vi "Force Array To Size.vi"(5 "Default Value":dbl format="%.2f", 6 "Boolean Array In":bool[](array[boolean]), 7 "# Elements":i32, 9 "2D U8 Array In":u8[][](array[numeric]), 10 "DBL Array In":dbl[](array[numeric]) format="%.2f", 11 "I32 Array In":i32[](array[numeric])) -> (1 "2D U8 Array Out":u8[][](array[numeric]), 2 "DBL Array Out":dbl[](array[numeric]) format="%.2f", 3 "I32 Array Out":i32[](array[numeric]), 4 "Boolean Array Out":bool[](array[boolean]))   [LabVIEW 2014]
panel:
  # "If input array has the specified number of elements, it is not changed.\nIf input array has more than the specified number of elements, the extra elements are removed from the end.\nIf input array has less than specified number of elements, it is padded using the default value."
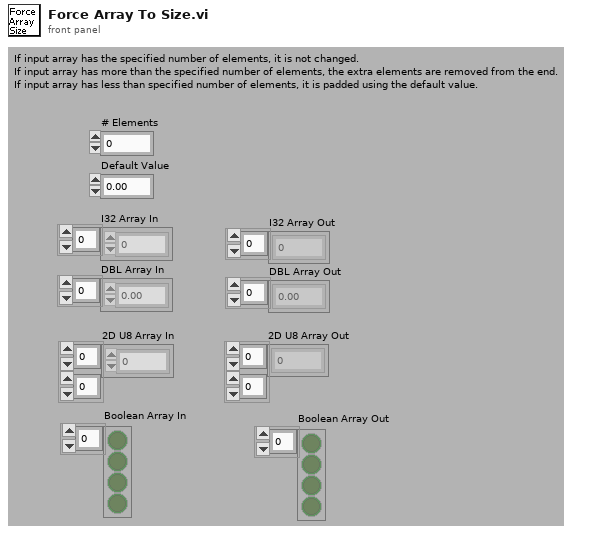
[diagram p1: front panel]
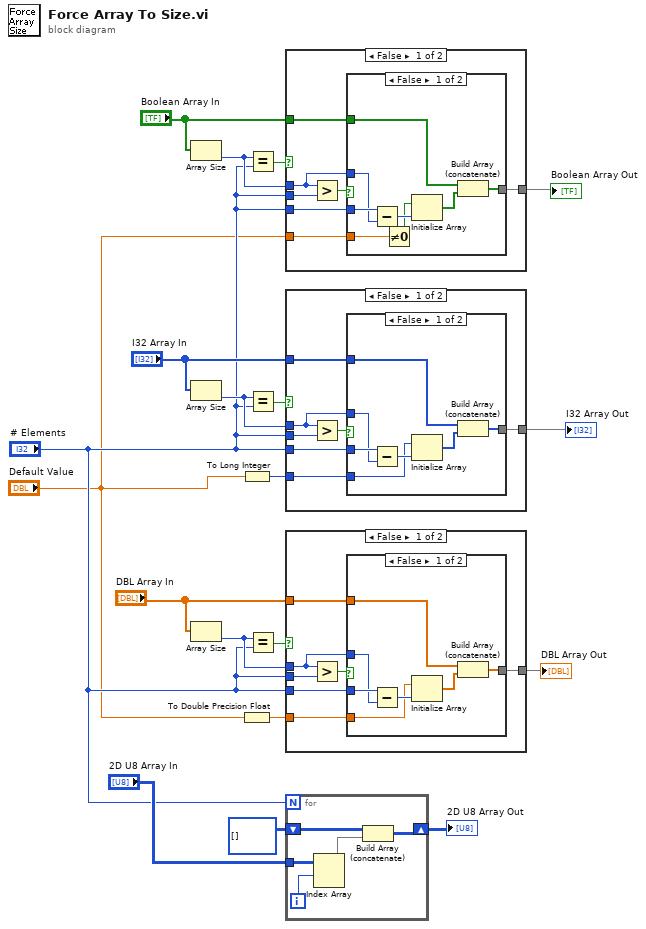
[diagram p0: block diagram]
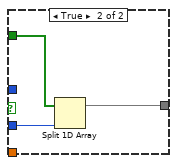
[diagram p2: hidden frame]
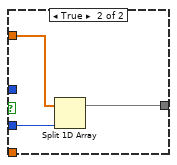
[diagram p4: hidden frame]
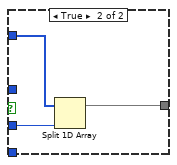
[diagram p6: hidden frame]
diagram:
  n1 = Array Size(array="Boolean Array In") -> (size(s)=w5:i32)
  n2 = Array Size(array="I32 Array In") -> (size(s)=w19:i32)
  n3 = Array Size(array="DBL Array In") -> (size(s)=w12:i32)
  n4 = To Long Integer(number="Default Value") -> (32bit integer=w16:i32)
  n5 = To Double Precision Float(number="Default Value") -> (double precision float=w14:dbl)
  n6 = Equal?(x=w5, y="# Elements") -> (x = y?=w6:bool)
  n7 = Equal?(x=w19, y="# Elements") -> (x = y?=w18:bool)
  n8 = Equal?(x=w12, y="# Elements") -> (x = y?=w13:bool)
  n9 = case shown="False" w6 {
    tunnel: w5 -> [w21 _]
    tunnel: "# Elements" -> [w26 _]
    tunnel: "# Elements" -> [w24 _]
    tunnel: "Boolean Array In" -> [w23 w38]
    tunnel: [w22 w38] -> w1
    tunnel: "Default Value" -> [w20 _]
    frame False {
      n10 = Greater?(x=w21, y=w26) -> (0:w25:bool)
      n11 = case shown="False" w25 {
        tunnel: w24 -> [w34 w37]
        tunnel: w23 -> [w30 w36]
        tunnel: [w29 w35] -> w22
        tunnel: w21 -> [w33 _]
        tunnel: w20 -> [w28 _]
        frame False {
          n12 = Subtract(x=w34, y=w33) -> (x-y=w32:i32)
          n13 = Not Equal To 0?(x=w28) -> (x != 0?=w27:bool)
          n14 = Initialize Array(w27, w32) -> (w31:bool[])
          n15 = Build Array (concatenate)(w30, w31) -> (w29:bool[])
        }
        frame True {
          n16 = Split 1D Array(array=w36, index=w37) -> (first subarray=w35:bool[])  [unwired: 1 out]
        }
      }
    }
    frame True {
    }
  }
  "Boolean Array Out" <- w1
  n17 = case shown="False" w18 {
    tunnel: w19 -> [w40 _]
    tunnel: "# Elements" -> [w45 _]
    tunnel: "# Elements" -> [w43 _]
    tunnel: "I32 Array In" -> [w42 w56]
    tunnel: [w41 w56] -> w15
    tunnel: w16 -> [w39 _]
    frame False {
      n18 = Greater?(x=w40, y=w45) -> (0:w44:bool)
      n19 = case shown="False" w44 {
        tunnel: w43 -> [w52 w55]
        tunnel: w42 -> [w47 w54]
        tunnel: [w46 w53] -> w41
        tunnel: w40 -> [w51 _]
        tunnel: w39 -> [w49 _]
        frame False {
          n20 = Subtract(x=w52, y=w51) -> (x-y=w50:i32)
          n21 = Initialize Array(w49, w50) -> (w48:i32[])
          n22 = Build Array (concatenate)(w47, w48) -> (w46:i32[])
        }
        frame True {
          n23 = Split 1D Array(array=w54, index=w55) -> (first subarray=w53:i32[])  [unwired: 1 out]
        }
      }
    }
    frame True {
    }
  }
  "I32 Array Out" <- w15
  n24 = case shown="False" w13 {
    tunnel: w12 -> [w58 _]
    tunnel: "# Elements" -> [w63 _]
    tunnel: "# Elements" -> [w61 _]
    tunnel: "DBL Array In" -> [w60 w74]
    tunnel: [w59 w74] -> w11
    tunnel: w14 -> [w57 _]
    frame False {
      n25 = Greater?(x=w58, y=w63) -> (0:w62:bool)
      n26 = case shown="False" w62 {
        tunnel: w61 -> [w70 w73]
        tunnel: w60 -> [w65 w72]
        tunnel: [w64 w71] -> w59
        tunnel: w58 -> [w69 _]
        tunnel: w57 -> [w67 _]
        frame False {
          n27 = Subtract(x=w70, y=w69) -> (x-y=w68:i32)
          n28 = Initialize Array(w67, w68) -> (w66:dbl[])
          n29 = Build Array (concatenate)(w65, w66) -> (w64:dbl[])
        }
        frame True {
          n30 = Split 1D Array(array=w72, index=w73) -> (first subarray=w71:dbl[])  [unwired: 1 out]
        }
      }
    }
    frame True {
    }
  }
  "DBL Array Out" <- w11
  n31 = for {
    N: "# Elements" -> [_]
    shift-right: [w75] -> w8
    shift-left: u8[][] [] -> [w76]
    tunnel: "2D U8 Array In" -> [w79]
    i -> [w78]
    n32 = Index Array(array=w79, index (row)=w78) -> (element=w77:u8[])  [unwired: 1 in]
    n33 = Build Array (concatenate)(w76, w77) -> (w75:u8[][])
  }
  "2D U8 Array Out" <- w8
